vi "Build Create.vi"(8 "error in (no error)":errorcluster, 9 "tableName":string, 10 "DynamicParameters in":refnum<class "DynamicParameters.lvclass">, 11 "SQLConnection in":refnum<class "DBC.lvclass">) -> (0 "error out":errorcluster, 1 "LastIdentityQuery":string, 2 "InsertStatement":string, 3 "SQLConnection out":refnum<class "DBC.lvclass">)   [LabVIEW 2020, in "ORM_DBC_Mssql.lvlib" / "DBC.lvclass"]
uses:
  DBC.lvclass
  <vilib>/Viviota/shared/ORM.lvlibp/ORM/DynamicParameters/DynamicParameters.lvclass
  <vilib>/Viviota/shared/ORM.lvlibp/ORM/DynamicParameters/Read AutoKey.vi
  <vilib>/Viviota/shared/ORM_DBC_dotNet.lvlibp/dbcDotNet/ORM_DBC_dotNet.lvclass
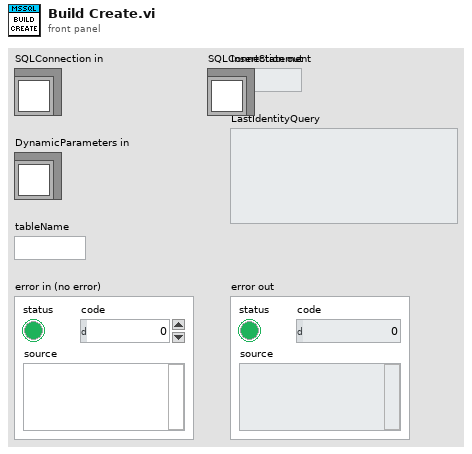
[diagram p1: front panel]
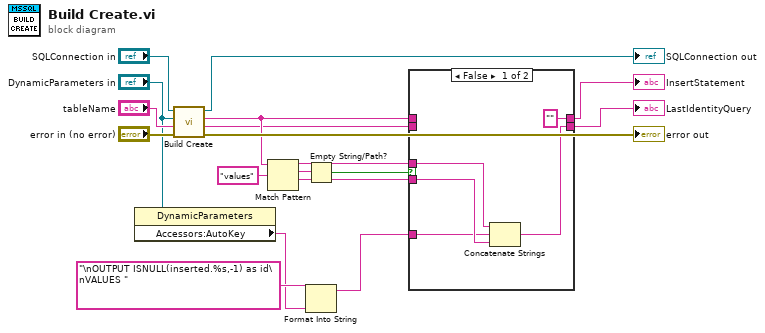
[diagram p0: block diagram]
diagram:
  n1 = property class="DynamicParameters"(reference="DynamicParameters in") -> ("Accessors:AutoKey"=w2:string)  [unwired: 1 in, 2 out]
  n2 = call-parent "Build Create.vi"("error in (no error)"="error in (no error)", "tableName"="tableName", "DynamicParameters in"="DynamicParameters in", "DbConnection in"="SQLConnection in") -> ("error out"=→"error out":errorcluster, "LastIdentityQuery"=w8:string, "InsertStatement"=w10:string, "DbConnection out"=→"SQLConnection out":refnum<class "DBC.lvclass">)  [unwired: 4 in]
  n3 = Match Pattern(string=w10, regular expression="values") -> (before substring=w6:string, match substring=w12:string, after substring=w5:string)  [unwired: 1 in, 1 out]
  n4 = Empty String/Path?(string/path=w12) -> (empty?=w11:bool)
  n5 = Format Into String(format string="\nOUTPUT ISNULL(inserted.%s,-1) as id\nVALUES " ("string"), w2) -> (resulting string=w1:string)  [unwired: 2 in, 1 out]
  n6 = case shown="False" w11 {
    tunnel: w10 -> [_ w25]
    tunnel: ["" ("InsertStatement") w25] -> w9
    tunnel: w8 -> [_ w24]
    tunnel: [w20 w24] -> w7
    tunnel: w6 -> [w21 _]
    tunnel: w5 -> [w23 _]
    tunnel: w1 -> [w22 _]
    frame False {
      n7 = Concatenate Strings(w21, w22, w23) -> (w20:string)
    }
    frame True {
    }
  }
  "LastIdentityQuery" <- w7
  "InsertStatement" <- w9
